vi "Pot init.vi"() -> (0 "AIDeviceRef":T1={"DevStatus"={"status"=FALSE, "code"=0, "source"=""}, "Analog Module"=enum."Analog Module 1", "Analog Channel"=enum."Invalid"})   [LabVIEW 2013]
uses:
  <vilib>/Rock Robotics/SystemInterfaces/Typedef/FPGA_TypedefAnalogModule.ctl
  <vilib>/Rock Robotics/SystemInterfaces/AI/FPGA_AIChannel.ctl
  <vilib>/Rock Robotics/WPI/AnalogChannel/WPI_AnalogChannelDevRef.ctl
panel:
  in  "Channel":T3=enum."AI 2"
  in  "Analog Module":T2
  in  "Samples Per Second":dbl=1000.0
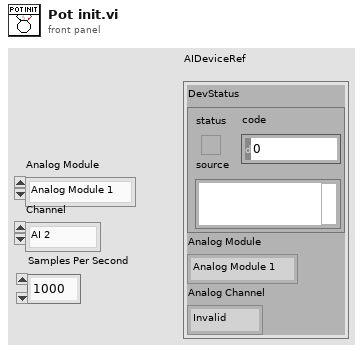
[diagram p1: front panel]
types:
  T1 = typedef "WPI_AnalogChannelDevRef.ctl" = cluster{"DevStatus":errorcluster, "Analog Module":T2, "Analog Channel":T3}
  T2 = typedef "FPGA_TypedefAnalogModule.ctl" = enum16{"Analog Module 1", "Analog Module 2"}
  T3 = typedef "FPGA_AIChannel.ctl" = enum8{"AI 1", "AI 2", "AI 3", "AI 4", "AI 5", "AI 6", "AI 7", "AI 8", "Invalid"}
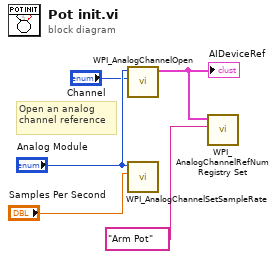
[diagram p0: block diagram]
diagram:
  # "Open an analog channel reference"
  n1 = call <vilib>:"WPI_AnalogChannelOpen.vi"("Analog Channel"="Channel", "Analog Module (Module 1)"="Analog Module") -> ("AIDeviceRef"=w2:T1)  [unwired: 1 in, 8 out]
  "AIDeviceRef" <- w2
  n2 = call <vilib>:"WPI_AnalogChannelSetSampleRate.vi"("Samples Per Second"="Samples Per Second", "Analog Module (Module 1)"="Analog Module") -> ()  [unwired: 2 in, 8 out]
  n3 = call <vilib>:"WPI_AnalogChannelRefNum Registry Set.vi"("refnum name"="Arm Pot", "AIDeviceRef"=w2) -> ()  [unwired: 8 in, 2 out]
